vi "Process.vi"(11 "Actor":refnum<class "About Window.lvclass">) -> ()   [LabVIEW 2015, in "About Window.lvclass"]
uses:
  About Window.lvclass
  Re-use Libraries/Utility/UI/System Button (without mouse hover).ctl
  Re-use Libraries/Minimal Actor Framework/Actors/Base Actor/Actor/Front Panel State.ctl
  Re-use Libraries/Minimal Actor Framework/Actors/Base Actor/Actor/Actor.lvclass
  Re-use Libraries/Minimal Actor Framework/Messaging/Message/Message.lvclass
  Actors/Alarm Handler/API/Alarm Handler Actor API.lvclass
  Re-use Libraries/Application Info/App Info.lvlib
  Actors/Main Controller/API/Main Controller Actor API.lvclass
  Re-use Libraries/Utility/Utility.lvlib
panel:
  in  "Close":T1
  out "Application Name 3":string
  in  "Boolean":bool
  out "Application Name":string
  # "Developed in LabVIEW.\nCopyright © 2018 National Instruments.\nAll rights reserved."
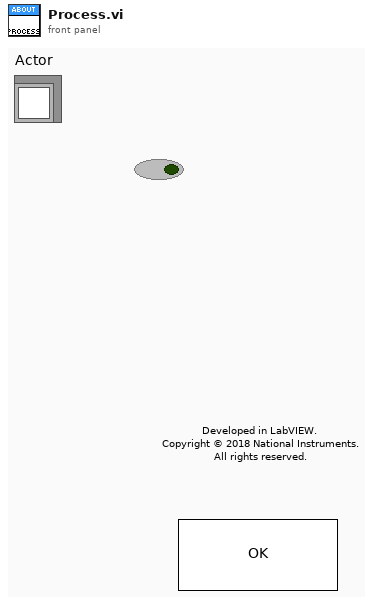
[diagram p1: front panel]
types:
  T1 = typedef "Utility.lvlib/System Button (without mouse hover).ctl" = bool
  T2 = typedef "Actor.lvclass/Front Panel State.ctl" = enum32{"Invalid", "Standard", "Closed", "Hidden", "Minimized", "Maximized"}
  T3 = typedef "App Info.lvlib/Core Data.ctl" = cluster{"Version":string, "Misc Info":string, "Name":string, "Name 2":string}
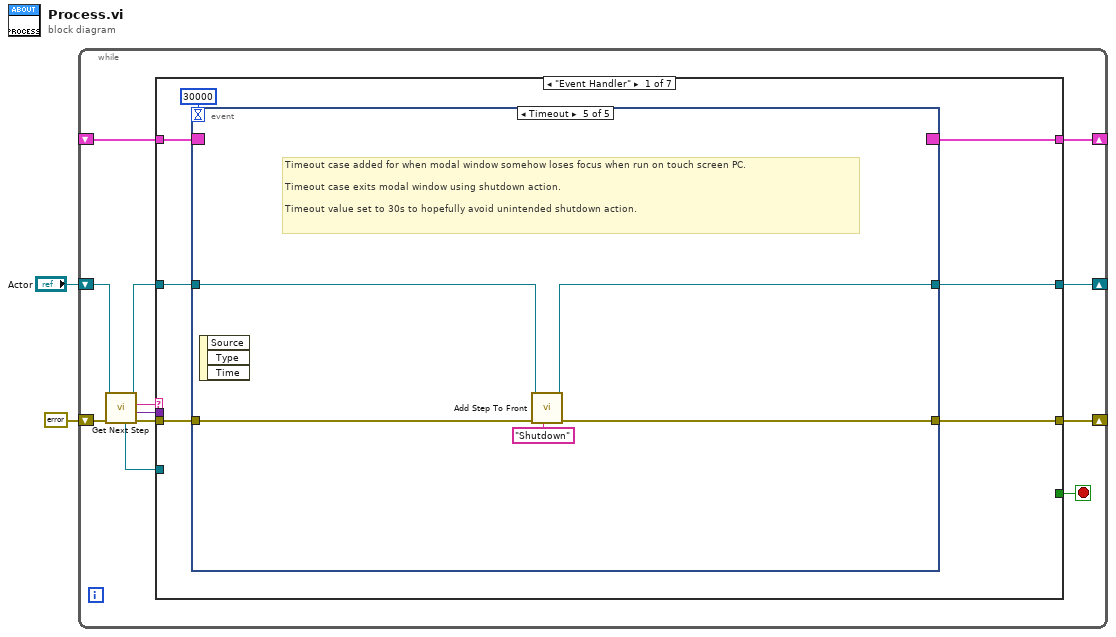
[diagram p0: block diagram]
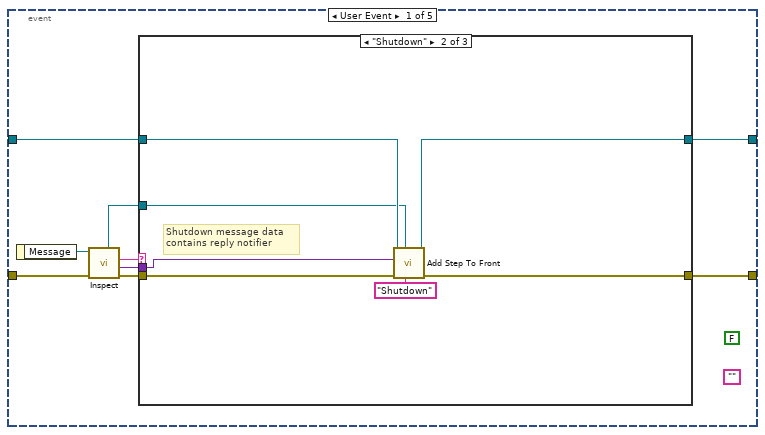
[diagram p2: hidden frame]
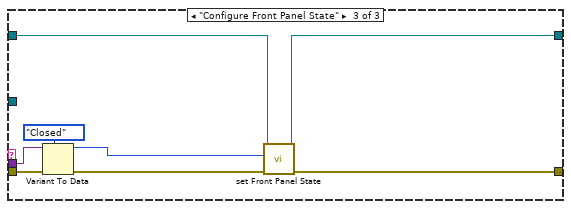
[diagram p4: hidden frame]
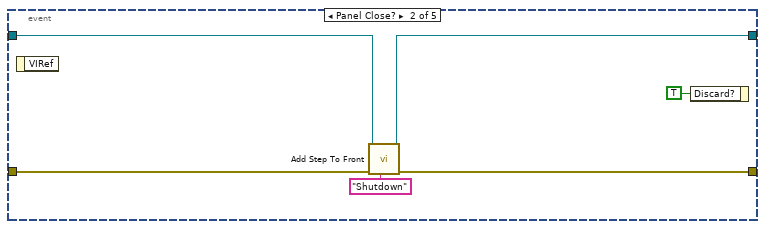
[diagram p5: hidden frame]
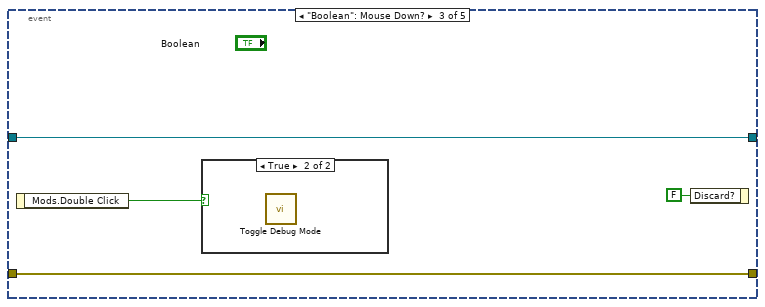
[diagram p6: hidden frame]
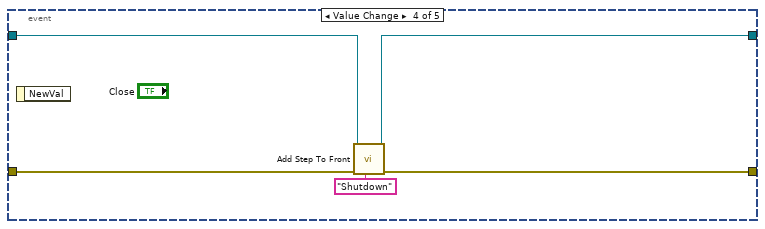
[diagram p8: hidden frame]
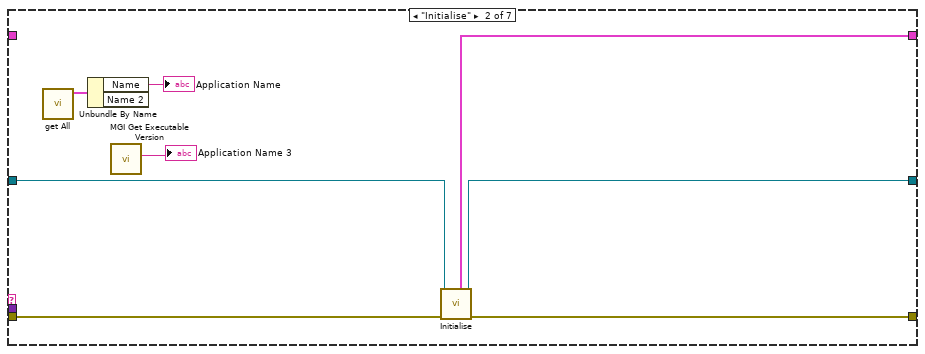
[diagram p9: hidden frame]
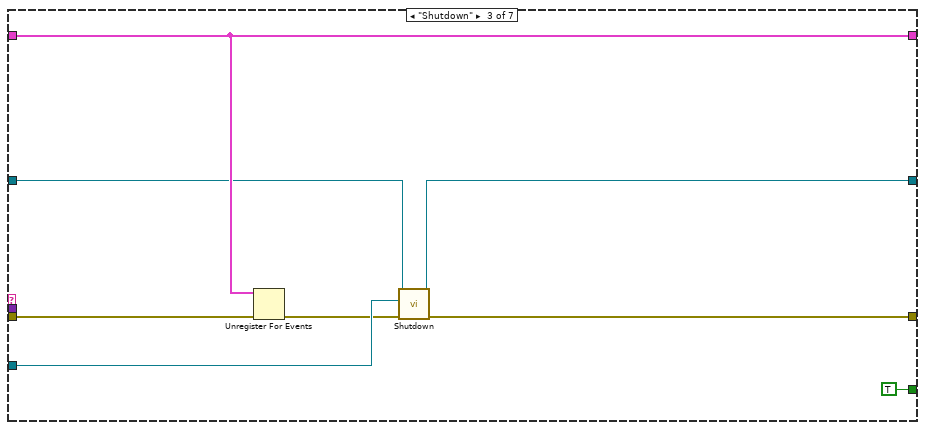
[diagram p10: hidden frame]
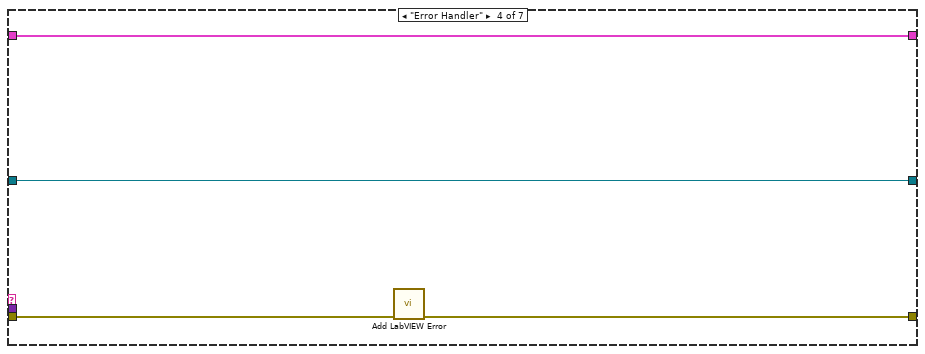
[diagram p11: hidden frame]
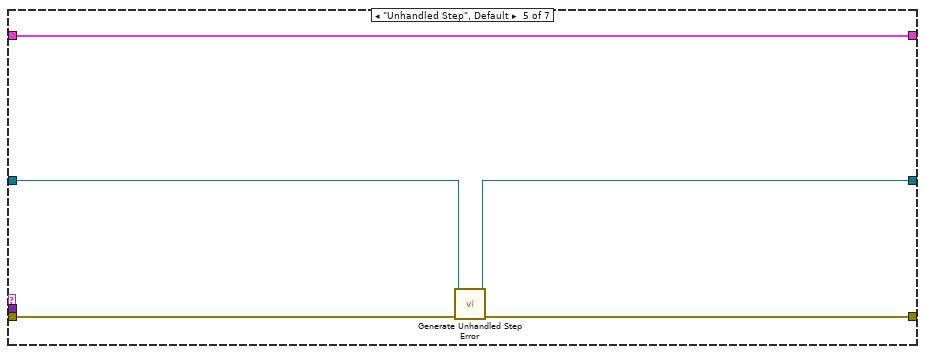
[diagram p12: hidden frame]
diagram:
  n1 = while {
    shift-right: [w5] -> _
    shift-left: "Actor" -> [w13]
    shift-right: [w10] -> _
    shift-left: _ -> [w9]
    shift-right: [w4] -> _
    shift-left: errorcluster {"status"=FALSE, "code"=0, "source"=""} ("error constant") -> [w7]
    stop <- w14 stop-if-true
    n2 = call-dynamic "Get Next Step.vi"("error in (no error)"=w7, "Actor in"=w13) -> ("error out"=w8:errorcluster, "Parameter"=w11:variant, "Step"=w6:string, "Actor out"=w12:refnum<class "About Window.lvclass">, "Reply Channel"=w3:refnum<notifier>)  [unwired: 5 in]
    n3 = case shown="\"Event Handler\"" w6 {
      tunnel: [_ _ TRUE _ _ _ _] -> w14
      tunnel: w12 -> [w21 w69 w81 w84 w91 w94 w96]
      tunnel: [w16 w74 w80 w84 w90 w94 w96] -> w5
      tunnel: w11 -> [_ _ _ _ _ _ _]
      tunnel: [w19 w75 w82 w87 w92 w95 w98] -> w10
      tunnel: w9 -> [w20 _ w82 w87 w92 w95 w98]
      tunnel: w8 -> [w18 w71 w78 w86 w89 w93 w97]
      tunnel: [w17 w70 w76 w85 w88 w93 w97] -> w4
      tunnel: w3 -> [_ _ w79 _ _ _ _]
      frame "Event Handler" {
        n4 = event shown="[4] Timeout" {
          selector: w20 -> [_ _ _ _ _]
          dyn-events: [_ _ _ _ _] -> w19
          timeout: 30000 -> [_ _ _ _ _]
          tunnel: w21 -> [w30 w49 w57 w61 w65]
          tunnel: [w29 w48 w57 w60 w64] -> w16
          tunnel: w18 -> [w27 w51 w54 w59 w66]
          tunnel: [w28 w50 w54 w58 w63] -> w17
          event User Event {
            (unwired) ""
            (unwired) FALSE
            n5 = event-data() -> ("Message"=w26:refnum<class "Message.lvclass">)  [unwired: 1 in]
            n6 = call "Inspect.vi"("error in (no error)"=w27, "Message in"=w26) -> ("error out"=w23:errorcluster, "Data"=w24:variant, "Name"=w25:string, "Reply Channel"=w22:refnum<notifier>)  [unwired: 5 in, 1 out]
            n7 = case shown="\"Shutdown\"" w25 {
              tunnel: w30 -> [w32 w39 w47]
              tunnel: [w32 w38 w46] -> w29
              tunnel: w23 -> [w31 w36 w43]
              tunnel: [w31 w35 w45] -> w28
              tunnel: w24 -> [_ w34 w44]
              tunnel: w22 -> [_ w33 _]
              frame Default {
              }
              frame "Shutdown" {
                # "Shutdown message data contains reply notifier"
                n8 = call-dynamic "Add Step To Front.vi"("Step Name"="Shutdown", "Reply Channel"=w33, "error in (no error)"=w36, "Parameter"=w34, "Actor in"=w39) -> ("error out"=w35:errorcluster, "Actor out"=w38:refnum<class "About Window.lvclass">)  [unwired: 5 in]
              }
              frame "Configure Front Panel State" {
                n9 = Variant To Data(error in=w43, type=Front_Panel_State."Closed" ("Front Panel State"), Variant=w44) -> (data=w40:T2, error out=w42:errorcluster)
                n10 = call-dynamic "set Front Panel State.vi"("error in (no error)"=w42, "Front Panel State"=w40, "Actor in"=w47) -> ("error out"=w45:errorcluster, "Actor out"=w46:refnum<class "About Window.lvclass">)  [unwired: 7 in]
              }
            }
          }
          event Panel Close? {
            n11 = event-data() -> ()  [unwired: 1 in, 1 out]
            n12 = call-dynamic "Add Step To Front.vi"("Step Name"="Shutdown", "error in (no error)"=w51, "Actor in"=w49) -> ("error out"=w50:errorcluster, "Actor out"=w48:refnum<class "About Window.lvclass">)  [unwired: 7 in]
            n13 = event-data("Discard?"=TRUE) -> ()  [unwired: 1 in, 1 out]
          }
          event "Boolean": Mouse Down? {
            n14 = event-data() -> ("Mods.Double Click"=w55:bool)  [unwired: 1 in]
            n15 = case shown="True" w55 {
              frame False {
              }
              frame True {
                n16 = call "Toggle Debug Mode.vi"() -> ()  [unwired: 11 in, 1 out]
              }
            }
            n17 = event-data("Discard?"=FALSE) -> ()  [unwired: 1 in, 1 out]
          }
          event Value Change {
            n18 = event-data() -> ()  [unwired: 1 in, 1 out]
            n19 = call-dynamic "Add Step To Front.vi"("Step Name"="Shutdown", "error in (no error)"=w59, "Actor in"=w61) -> ("error out"=w58:errorcluster, "Actor out"=w60:refnum<class "About Window.lvclass">)  [unwired: 7 in]
          }
          event Timeout {
            # "Timeout case added for when modal window somehow loses focus when run on touch screen PC.\n\nTimeout case exits modal window using shutdown action.\n\nTimeout value set to 30s to hopefully avoid unintended shutdown action."
            n20 = event-data() -> ()  [unwired: 1 in, 3 out]
            n21 = call-dynamic "Add Step To Front.vi"("Step Name"="Shutdown", "error in (no error)"=w66, "Actor in"=w65) -> ("error out"=w63:errorcluster, "Actor out"=w64:refnum<class "About Window.lvclass">)  [unwired: 7 in]
          }
        }
      }
      frame "Initialise" {
        n22 = call "get All.vi"() -> ("Data out"=w72:T3)  [unwired: 10 in, 1 out]
        n23 = Unbundle By Name(w72) -> ("Name"=→"Application Name":string)  [unwired: 1 out]
        n24 = call <userlib>:"MGI Get Executable Version.vi"() -> ("Version"=→"Application Name 3":string)  [unwired: 7 in]
        n25 = call "Initialise.vi"("error in (no error)"=w71, "Actor in"=w69) -> ("error out"=w70:errorcluster, "Actor out"=w74:refnum<class "About Window.lvclass">, "Observers"=w75:cluster{"Actor":refnum<event-registration>})  [unwired: 7 in]
      }
      frame "Shutdown" {
        n26 = Unregister For Events(event registration refnum=w82, error in=w78) -> (error out=w77:errorcluster)
        n27 = call-dynamic "Shutdown.vi"("error in (no error)"=w77, "Reply Channel"=w79, "Actor in"=w81) -> ("error out"=w76:errorcluster, "Actor out"=w80:refnum<class "About Window.lvclass">)  [unwired: 7 in]
      }
      frame "Error Handler" {
        n28 = call "Add LabVIEW Error.vi"("error in (no error)"=w86) -> ("error out"=w85:errorcluster)  [unwired: 10 in]
      }
      frame "Unhandled Step", Default {
        n29 = call-dynamic "Generate Unhandled Step Error.vi"("error in (no error)"=w89, "Actor in"=w91) -> ("error out"=w88:errorcluster, "Actor out"=w90:refnum<class "About Window.lvclass">)  [unwired: 8 in]
      }
      frame "-----------------------" {
        # "Separator"
      }
      frame "Update State" {
        # "Not used"
      }
    }
  }
